vi "Wavelength Limiter.vi"(4 "Range Limiter(F) or WL limiter":bool, 5 "Current Grating Density":T3=enum."1200" caption="Grating Density", 7 "Central WL Input":dbl=619.92122 format="%.4f", 8 "X-Axis":T2=enum."nm") -> (0 "Wavelength Range":T1 {"Increment" format="%.2f"; "Maximum" format="%.2f"; "Minimum" format="%.2f"}, 1 "Maximum Value":dbl=619.92122 format="%.4f", 2 "Central WL output":dbl=619.92122 caption="Central WL Output" format="%.4f", 3 "Minimum Value":dbl=619.92122 format="%.4f")   [LabVIEW 2020]
uses:
  Globals and TypeDefs/Type Definitions.llb/McPherson Grating Density.ctl
  Globals and TypeDefs/Type Definitions.llb/Wavelength Unit.ctt
  File and save/X-Axis Converter.llb/X-Axis Converter.vi
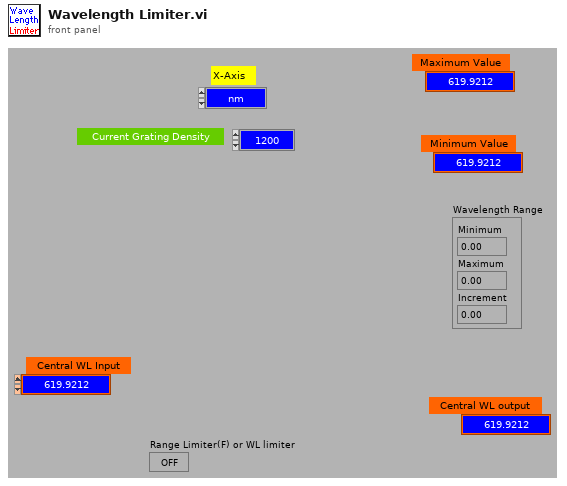
[diagram p1: front panel]
types:
  T1 = cluster{"Minimum":dbl, "Maximum":dbl, "Increment":dbl}
  T2 = typedef "Wavelength Unit.ctt" = enum8{"Point", "nm", "eV", "meV", "cm_1"}
  T3 = typedef "McPherson Grating Density.ctl" = enum8{"150", "300", "600", "1200", "1800"}
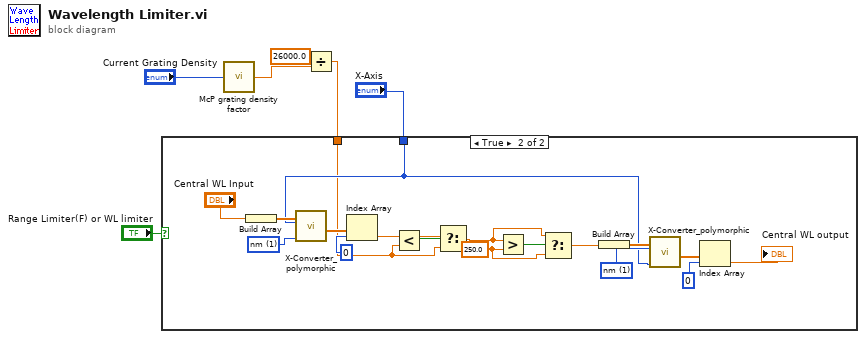
[diagram p0: block diagram]
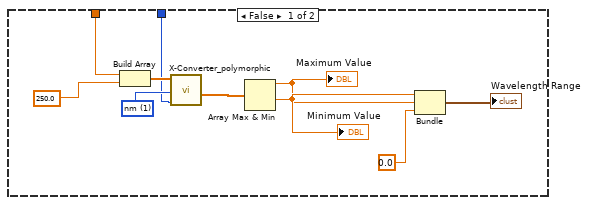
[diagram p2: hidden frame]
diagram:
  n1 = call "McP grating density factor.vi"("Grating Density"="Current Grating Density") -> ("GratingFactor"=w3:dbl)
  n2 = Divide(x=26000.0, y=w3) -> (x/y=w2:dbl)
  n3 = case shown="True" "Range Limiter(F) or WL limiter" {
    tunnel: "X-Axis" -> [w8 w18]
    tunnel: w2 -> [w7 w17]
    frame False {
      w15 = 1 items=["Point #", "nm", "eV", "meV", "cm-1"] ("X-Axis Unit")
      n4 = Build Array(w7, 250.0 ("y")) -> (w16:dbl[])
      n5 = call-poly "X-Converter_polymorphic.vi"("X-Axis Unit"=w8, "Old X-Axis Unit"=w15, "X-Axis input"=w16) -> ("X-Axis Output"=w13:dbl[])  [unwired: 2 in, 3 out]
      n6 = Array Max & Min(array=w13) -> (max value=w9:dbl, min value=w10:dbl)  [unwired: 2 out]
      "Maximum Value" <- w9
      "Minimum Value" <- w10
      n7 = Bundle(w10, w9, "y"=0.0) -> (→"Wavelength Range":cluster{dbl, dbl, "y":dbl})  [unwired: 1 in]
    }
    frame True {
      w21 = 1 items=["Point #", "nm", "eV", "meV", "cm-1"] ("X-Axis Unit")
      w28 = 1 items=["Point #", "nm", "eV", "meV", "cm-1"] ("X-Axis Unit")
      w31 = 250.0 ("y")
      n8 = Build Array("Central WL Input") -> (w20:dbl[])
      n9 = call-poly "X-Converter_polymorphic.vi"("X-Axis Unit"=w21, "Old X-Axis Unit"=w18, "X-Axis input"=w20) -> ("X-Axis Output"=w22:dbl[])  [unwired: 2 in, 3 out]
      n10 = Index Array(array=w22, index=0) -> (element=w25:dbl)
      n11 = Less?(x=w25, y=w17) -> (x < y?=w24:bool)
      n12 = Select(t=w25, s=w24, f=w17) -> (s? t:f=w30:dbl)
      n13 = Greater?(x=w30, y=w31) -> (0:w29:bool)
      n14 = Select(t=w30, s=w29, f=w31) -> (s? t:f=w32:dbl)
      n15 = Build Array(w32) -> (w26:dbl[])
      n16 = call-poly "X-Converter_polymorphic.vi"("X-Axis Unit"=w18, "Old X-Axis Unit"=w28, "X-Axis input"=w26) -> ("X-Axis Output"=w27:dbl[])  [unwired: 2 in, 3 out]
      n17 = Index Array(array=w27, index=0) -> (element=→"Central WL output":dbl)
    }
  }
